vi "Get HLAfloat64BE.vi"(11 "raw data in":u8[](array[numeric])) -> (1 "valid":bool=TRUE, 3 "eu data out":dbl[](array[numeric]))   [LabVIEW 2019, in "HLA Data Conversion.lvlib"]
uses:
  HLA Data Conversion.lvlib
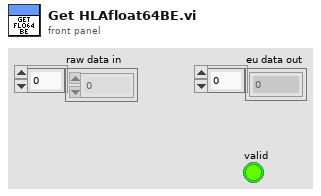
[diagram p1: front panel]
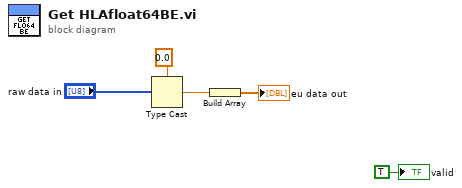
[diagram p0: block diagram]
diagram:
  n1 = Type Cast(type=0.0 ("world.location.x"), x="raw data in") -> (*(type *) &x=w3:dbl)
  n2 = Build Array(w3) -> (→"eu data out":dbl[])
  "valid" <- TRUE
